vi "Compute SRAD Filter 32f.vi"(8 "Error In":errorcluster, 9 "Data In":sgl[][][](array[numeric]), 10 "SRAD Filter Options":T8, 11 "Anisotropic Filter Object":T1={"Device In"=0, "Program Handle"=0, "N"={"Device ID"=0, "Memeroy ID"=0, "Dimension"={"Depth"=0, "Height"=0, "Width"=0}, "Memory Type"=enum."32f"}, "N + 1"={"Device ID"=0, "Memeroy ID"=0, "Dimension"={"Depth"=0, "Height"=0, "Width"=0}, "Memory Type"=enum."32f"}, "Dimensions"={"Depth"=1, "Height"=1, "Width"=1}, "Diffusivity"={"Device ID"=0, "Memeroy ID"=0, "Dimension"={"Depth"=0, "Height"=0, "Width"=0}, "Memory Type"=enum."32f"}} {"Diffusivity"."Dimension"."Width" min=1; "Diffusivity"."Dimension"."Height" min=1; "Diffusivity"."Dimension"."Depth" min=1; "Dimensions"."Width" min=1; "Dimensions"."Height" min=1; "Dimensions"."Depth" min=1; "N + 1"."Dimension"."Width" min=1; "N + 1"."Dimension"."Height" min=1; "N + 1"."Dimension"."Depth" min=1; "N"."Dimension"."Width" min=1; "N"."Dimension"."Height" min=1; "N"."Dimension"."Depth" min=1}) -> (0 "Error Out":errorcluster, 2 "Data Out":sgl[][][](array[numeric]), 3 "Anisotropic Filter Object Out":T1={"Device In"=0, "Program Handle"=0, "N"={"Device ID"=0, "Memeroy ID"=0, "Dimension"={"Depth"=0, "Height"=0, "Width"=0}, "Memory Type"=enum."32f"}, "N + 1"={"Device ID"=0, "Memeroy ID"=0, "Dimension"={"Depth"=0, "Height"=0, "Width"=0}, "Memory Type"=enum."32f"}, "Dimensions"={"Depth"=1, "Height"=1, "Width"=1}, "Diffusivity"={"Device ID"=0, "Memeroy ID"=0, "Dimension"={"Depth"=0, "Height"=0, "Width"=0}, "Memory Type"=enum."32f"}} {"Diffusivity"."Dimension"."Width" min=1; "Diffusivity"."Dimension"."Height" min=1; "Diffusivity"."Dimension"."Depth" min=1; "Dimensions"."Width" min=1; "Dimensions"."Height" min=1; "Dimensions"."Depth" min=1; "N + 1"."Dimension"."Width" min=1; "N + 1"."Dimension"."Height" min=1; "N + 1"."Dimension"."Depth" min=1; "N"."Dimension"."Width" min=1; "N"."Dimension"."Height" min=1; "N"."Dimension"."Depth" min=1}, 4 "Time in ms":dbl)   [LabVIEW 2012, in "OpenCLV x64.lvlib"]
doc: "Speckle Reducing Anisotropic Diffusion Filter from Bovik \"Essential Guide to Image Processing\" chapter 20.3.6"
uses:
  OpenCLV x64.lvlib
  Controls/SRAD Filter Object.ctl
  Controls/Device ID.ctl
  Controls/Program Handle.ctl
  Controls/Memory Object.ctl
  Controls/Memory ID.ctl
  Controls/Memory Type.ctl
  Controls/SRAD Filter Options.ctl
  Write Memory/WriteMemory_32f.vi
  Read Memory/ReadMemory_32f.vi
  Set Kernel Arguments/Set Kernel Arguments Memory Object.vi
  Set Kernel Arguments/Set Kernel Arguments 32f.vi
  User Controls/Array Dimensions.ctl
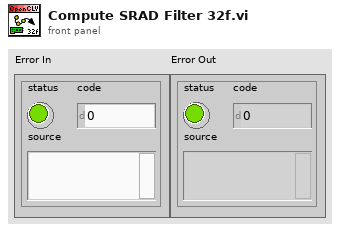
[diagram p1: front panel]
types:
  T1 = typedef "OpenCLV x64.lvlib/SRAD Filter Object.ctl" = cluster{"Device In":T2, "Program Handle":T3, "N":T4, "N + 1":T4, "Dimensions":T6, "Diffusivity":T4}
  T2 = typedef "OpenCLV x64.lvlib/Device ID.ctl" = u64
  T3 = typedef "OpenCLV x64.lvlib/Program Handle.ctl" = u64
  T4 = typedef "OpenCLV x64.lvlib/Memory Object.ctl" = cluster{"Device ID":T2, "Memeroy ID":T5, "Dimension":T6, "Memory Type":T7}
  T5 = typedef "OpenCLV x64.lvlib/Memory ID.ctl" = u64
  T6 = typedef "Array Dimensions.ctl" = cluster{"Depth":u64, "Height":u64, "Width":u64}
  T7 = typedef "OpenCLV x64.lvlib/Memory Type.ctl" = enum16{"32f", "u8", "i8", "u16", "i16", "u32", "i32", "64f"}
  T8 = typedef "OpenCLV x64.lvlib/SRAD Filter Options.ctl" = cluster{"Threshold":dbl, "Step Time":dbl, "Total Time":dbl}
  T9 = typedef "OpenCLV x64.lvlib/Kernel Handle.ctl" = u64
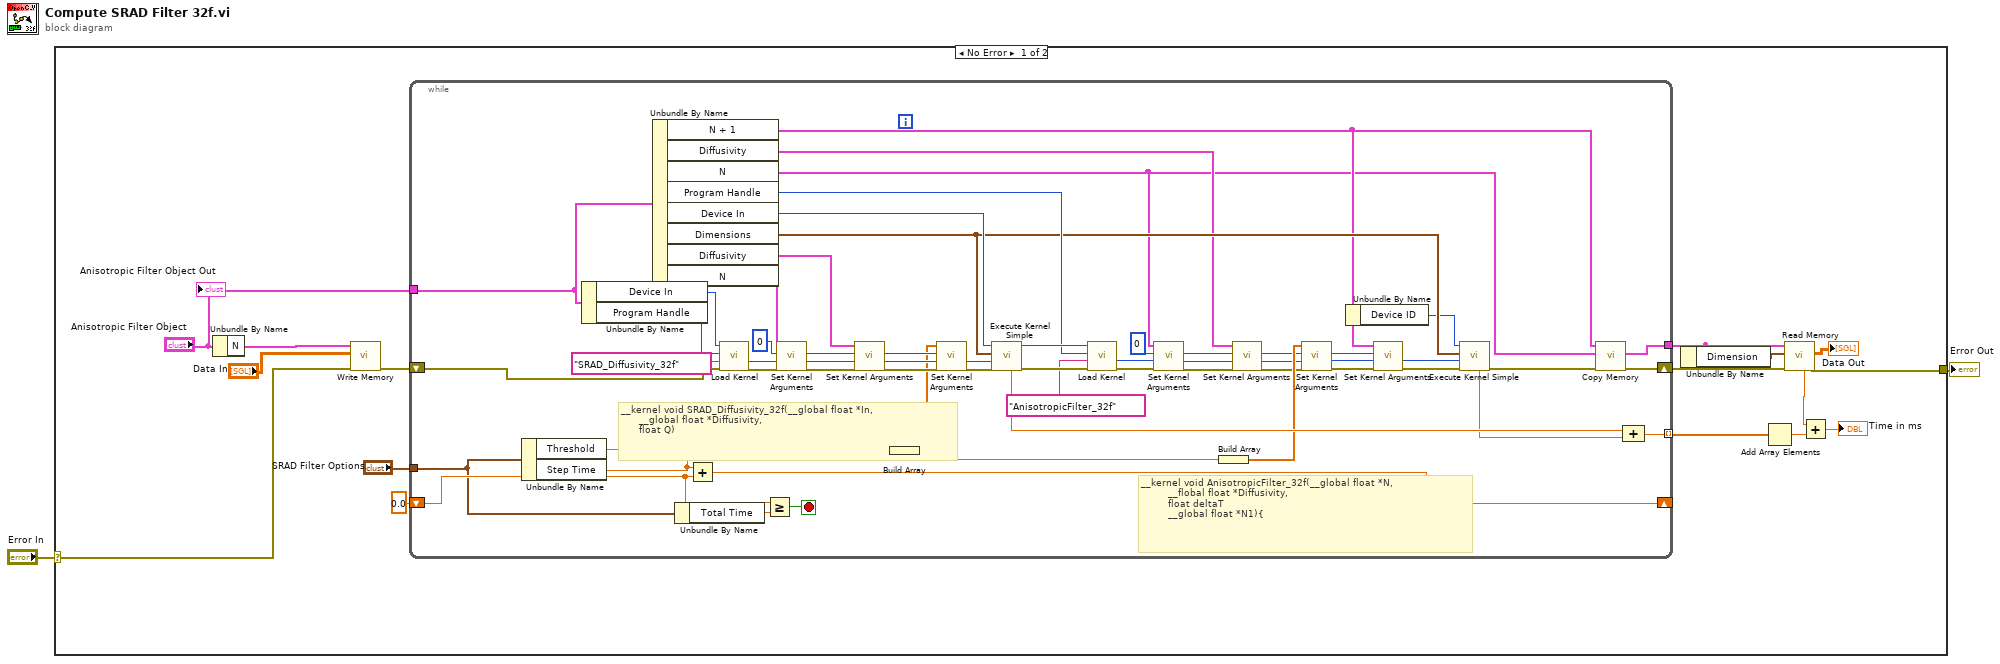
[diagram p0: block diagram]
diagram:
  n1 = case shown="No Error" "Error In" {
    selector: "Error In" -> [w10 w76]
    tunnel: [w17 w76] -> w2
    frame No Error {
      n2 = Unbundle By Name("Anisotropic Filter Object") -> ("N"=w7:T4)
      n3 = call-poly "Write Memory.vi"("Error In"=w10, "Data In"="Data In", "Memory Object In"=w7) -> ("Error Out"=w12:errorcluster)  [unwired: 6 in, 2 out]
      n4 = while {
        tunnel: "Anisotropic Filter Object" -> [w56]
        shift-right: [w57] -> w18
        shift-left: w12 -> [w52]
        tunnel: [w20] -> w4
        tunnel: [w62] -> w16 mode=indexing
        shift-right: [w60] -> _
        shift-left: sgl 0.0 -> [w58]
        tunnel: "SRAD Filter Options" -> [w47]
        stop <- w59 stop-if-true
        # "__kernel void SRAD_Diffusivity_32f(__global float *In, \n\t\t\t   __global float *Diffusivity,\n\t\t\t   float Q)"
        # "__kernel void AnisotropicFilter_32f(__global float *N,\n\t\t\t\t\t\t\t\t\t__flobal float *Diffusivity,\n\t\t\t\t\t\t\t\t\tfloat deltaT\n\t\t\t\t\t\t\t\t\t__global float *N1){"
        n5 = Unbundle By Name(w47) -> ("Threshold"=w45:dbl, "Step Time"=w43:dbl)
        n6 = Unbundle By Name(w56) -> ("Device In"=w75:T2, "Program Handle"=w74:T3)
        n7 = Unbundle By Name(w56) -> ("N + 1"=w37:T4, "Diffusivity"=w21:T4, "N"=w19:T4, "Program Handle"=w48:T3, "Device In"=w53:T2, "Dimensions"=w42:T6, "Diffusivity"=w38:T4, "N"=w39:T4)
        n8 = Unbundle By Name(w47) -> ("Total Time"=w61:dbl)
        n9 = Add(x=w43, y=w58) -> (x+y=w60:dbl)
        n10 = call "Load Kernel.vi"("Error In"=w52, "Kernel Name"="SRAD_Diffusivity_32f", "Program Handle"=w74, "Device In"=w75) -> ("Error Out"=w71:errorcluster, "Kernel Handle"=w72:T9)  [unwired: 4 in, 2 out]
        n11 = Greater Or Equal?(x=w58, y=w61) -> (x >= y?=w59:bool)
        n12 = call-poly "Set Kernel Arguments.vi"("Error In"=w71, "Kernel Handle"=w72, "Argument Number"=0, "Memory Object"=w39) -> ("Error Out"=w69:errorcluster, "Kernel Handle out"=w68:T9, "Auto Inc Arugment Number"=w67:i32)  [unwired: 5 in]
        n13 = call-poly "Set Kernel Arguments.vi"("Error In"=w69, "Kernel Handle"=w68, "Argument Number"=w67, "Memory Object"=w38) -> ("Error Out"=w66:errorcluster, "Kernel Handle out"=w65:T9, "Auto Inc Arugment Number"=w64:i32)  [unwired: 5 in]
        n14 = Build Array(w45) -> (w46:dbl[])
        n15 = call-poly "Set Kernel Arguments.vi"("Error In"=w66, "Kernel Handle"=w65, "Argument Number"=w64, "32f Constant"=w46) -> ("Error Out"=w54:errorcluster, "Kernel Handle out"=w55:T9)  [unwired: 5 in, 1 out]
        n16 = call "Execute Kernel Simple.vi"("Error In"=w54, "Kernel Handle"=w55, "Thread Dimensions"=w42, "Device In"=w53) -> ("Error Out"=w51:errorcluster, "Device Out"=w49:T2, "Time in ms"=w63:dbl)  [unwired: 4 in, 1 out]
        n17 = call "Load Kernel.vi"("Error In"=w51, "Kernel Name"="AnisotropicFilter_32f", "Program Handle"=w48, "Device In"=w49) -> ("Error Out"=w30:errorcluster, "Kernel Handle"=w26:T9)  [unwired: 4 in, 2 out]
        n18 = call-poly "Set Kernel Arguments.vi"("Error In"=w30, "Kernel Handle"=w26, "Argument Number"=0, "Memory Object"=w19) -> ("Error Out"=w31:errorcluster, "Kernel Handle out"=w32:T9, "Auto Inc Arugment Number"=w33:i32)  [unwired: 5 in]
        n19 = Build Array(w43) -> (w44:dbl[])
        n20 = call-poly "Set Kernel Arguments.vi"("Error In"=w31, "Kernel Handle"=w32, "Argument Number"=w33, "Memory Object"=w21) -> ("Error Out"=w34:errorcluster, "Kernel Handle out"=w35:T9, "Auto Inc Arugment Number"=w36:i32)  [unwired: 5 in]
        n21 = call-poly "Set Kernel Arguments.vi"("Error In"=w34, "Kernel Handle"=w35, "Argument Number"=w36, "32f Constant"=w44) -> ("Error Out"=w29:errorcluster, "Kernel Handle out"=w28:T9, "Auto Inc Arugment Number"=w27:i32)  [unwired: 5 in]
        n22 = Unbundle By Name(w37) -> ("Device ID"=w22:T2)
        n23 = call-poly "Set Kernel Arguments.vi"("Error In"=w29, "Kernel Handle"=w28, "Argument Number"=w27, "Memory Object"=w37) -> ("Error Out"=w24:errorcluster, "Kernel Handle out"=w23:T9)  [unwired: 5 in, 1 out]
        n24 = call "Execute Kernel Simple.vi"("Error In"=w24, "Kernel Handle"=w23, "Thread Dimensions"=w42, "Device In"=w22) -> ("Error Out"=w41:errorcluster, "Time in ms"=w40:dbl)  [unwired: 4 in, 2 out]
        n25 = call "Copy Memory.vi"("Error In"=w41, "Destination Object"=w19, "Source Object"=w37) -> ("Error Out"=w57:errorcluster, "Destination Object Out"=w20:T4)  [unwired: 6 in, 1 out]
        n26 = Compound Arithmetic op=ADD(w63, w40) -> (w62:dbl)
      }
      n27 = Unbundle By Name(w4) -> ("Dimension"=w3:T6)
      n28 = Add Array Elements(numeric array=w16) -> (sum=w15:dbl)
      n29 = call-poly "Read Memory.vi"("Error In"=w18, "Dimensions"=w3, "Memory Object In"=w4) -> ("Error Out"=w17:errorcluster, "Data Out"=→"Data Out":sgl[][][], "ms"=w14:dbl)  [unwired: 5 in, 1 out]
      n30 = Add(x=w14, y=w15) -> (x+y=→"Time in ms":dbl)
      "Anisotropic Filter Object Out" <- "Anisotropic Filter Object"
    }
    frame Error {
    }
  }
  "Error Out" <- w2
